vi "LOC subReadWriteVIStringINIKeys(VITitle).vi"(4 "Mode":enum16{"Read", "Write"}(ring), 5 "VIName":string, 6 "error in (no error)":errorcluster, 8 "ConfigFileRefnum":T1, 9 "VIRefnum":refnum<vi>) -> (0 "error out":errorcluster, 3 "dup VIRefnum":refnum<vi>)   [LabVIEW 2020, in "Localization_Tools.lvlib"]
uses:
  Localization_Tools.lvlib
  <vilib>/Utility/config.llb/Config Data RefNum.ctl
  <vilib>/Utility/config.llb/NI_LVConfig.lvlib
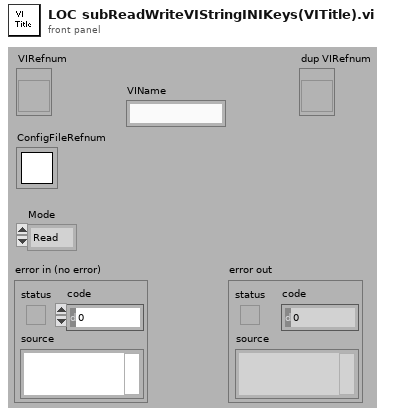
[diagram p1: front panel]
types:
  T1 = typedef "NI_LVConfig.lvlib/Config Data RefNum.ctl" = refnum<k1>
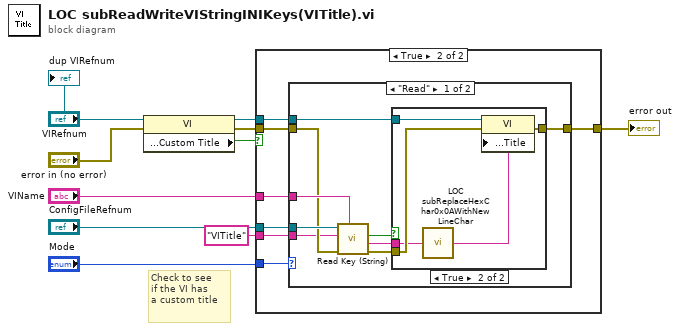
[diagram p0: block diagram]
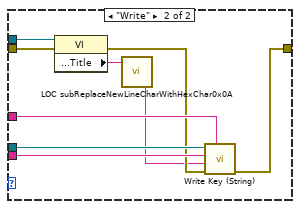
[diagram p4: hidden frame]
diagram:
  # "Check to see\nif the VI has\na custom title"
  n1 = property class="VI"(reference="VIRefnum", error in="error in (no error)") -> (reference out=w10:refnum<vi>, error out=w9:errorcluster, "Front Panel Window:Custom Title"=w1:bool)
  n2 = case shown="True" w1 {
    tunnel: w10 -> [_ w18]
    tunnel: w9 -> [w11 w17]
    tunnel: "Mode" -> [_ w16]
    tunnel: "ConfigFileRefnum" -> [_ w15]
    tunnel: "VIName" -> [_ w14]
    tunnel: "VITitle" ("key") -> [_ w13]
    tunnel: [w11 w12] -> w3
    frame False {
      # "For non-UI VIs, they will not have a custom title\nso do nothing."
    }
    frame True {
      n3 = case shown="\"Read\"" w16 {
        tunnel: w18 -> [w25 w42]
        tunnel: w17 -> [w23 w41]
        tunnel: w15 -> [w27 w40]
        tunnel: w14 -> [w26 w38]
        tunnel: w13 -> [w22 w39]
        tunnel: [w21 w36] -> w12
        frame "Read" {
          n4 = call <vilib>:"Read Key (String).vi"("section"=w26, "error in (no error)"=w23, "key"=w22, "refnum"=w27) -> ("error out"=w24:errorcluster, "value"=w20:string, "found?"=w19:bool)  [unwired: 4 in, 1 out]
          n5 = case shown="True" w19 {
            tunnel: w25 -> [_ w33]
            tunnel: w24 -> [w28 w32]
            tunnel: [w28 w31] -> w21
            tunnel: w20 -> [_ w30]
            frame False {
            }
            frame True {
              n6 = call "LOC subReplaceHexChar0x0AWithNewLineChar.vi"("InputString"=w30) -> ("OutputString"=w29:string)
              n7 = property class="VI"(reference=w33, error in=w32, "Front Panel Window:Title"=w29) -> (error out=w31:errorcluster)  [unwired: 1 out]
            }
          }
        }
        frame "Write" {
          n8 = property class="VI"(reference=w42, error in=w41) -> (error out=w37:errorcluster, "Front Panel Window:Title"=w34:string)  [unwired: 1 out]
          n9 = call "LOC subReplaceNewLineCharWithHexChar0x0A.vi"("InputString"=w34) -> ("OutputString"=w35:string)
          n10 = call <vilib>:"Write Key (String).vi"("section"=w38, "error in (no error)"=w37, "value"=w35, "key"=w39, "refnum"=w40) -> ("error out"=w36:errorcluster)  [unwired: 4 in, 2 out]
        }
      }
    }
  }
  "error out" <- w3
  "dup VIRefnum" <- "VIRefnum"
